vi "test_rigol_read_ascii.vi"() -> ()   [LabVIEW 2018]
panel:
  in  "VISA resource name":refnum<visa-resource-name>
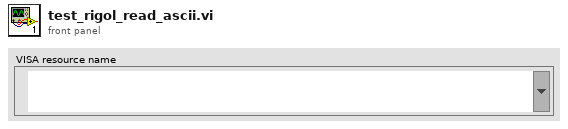
[diagram p1: front panel]
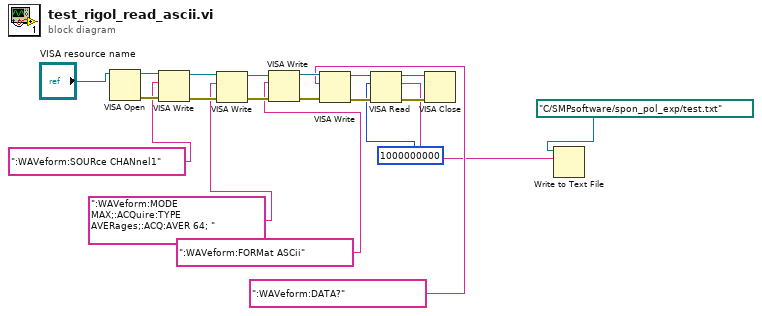
[diagram p0: block diagram]
diagram:
  n1 = VISA Open(VISA resource name="VISA resource name") -> (VISA resource name=w17:refnum<visa-resource-name>, error out=w16:errorcluster)  [unwired: 4 in]
  n2 = VISA Write(VISA resource name=w17, write buffer=":WAVeform:SOURce CHANnel1", error in (no error)=w16) -> (VISA resource name out=w14:refnum<visa-resource-name>, error out=w15:errorcluster)  [unwired: 1 out]
  n3 = VISA Write(VISA resource name=w14, write buffer=":WAVeform:MODE MAX;:ACQuire:TYPE AVERages;:ACQ:AVER 64; ", error in (no error)=w15) -> (VISA resource name out=w13:refnum<visa-resource-name>, error out=w12:errorcluster)  [unwired: 1 out]
  n4 = VISA Write(VISA resource name=w13, write buffer=":WAVeform:FORMat ASCii", error in (no error)=w12) -> (VISA resource name out=w11:refnum<visa-resource-name>, error out=w10:errorcluster)  [unwired: 1 out]
  n5 = VISA Write(VISA resource name=w11, write buffer=":WAVeform:DATA?", error in (no error)=w10) -> (VISA resource name out=w9:refnum<visa-resource-name>, error out=w8:errorcluster)  [unwired: 1 out]
  n6 = VISA Read(VISA resource name=w9, byte count=1000000000, error in (no error)=w8) -> (VISA resource name out=w18:refnum<visa-resource-name>, read buffer=w2:string, error out=w19:errorcluster)  [unwired: 1 out]
  n7 = VISA Close(VISA resource name=w18, error in (no error)=w19) -> ()  [unwired: 1 out]
  n8 = Write to Text File(file (use dialog)=path "C:/SMPsoftware/spon_pol_exp/test.txt", text=w2) -> ()  [unwired: 2 in, 3 out]
